vi "command move.vi"(8 "error in (no error)":errorcluster, 9 "uPosition":i32, 10 "Position":i32, 11 "id":i32) -> (0 "error out":errorcluster, 3 "function return":i32)   [LabVIEW 2020, in "libximc.lvlib"]
doc: "result_t XIMC_API command_move (device_t id, int Position, int uPosition);"
uses:
  libximc.lvlib
  libximc.dll
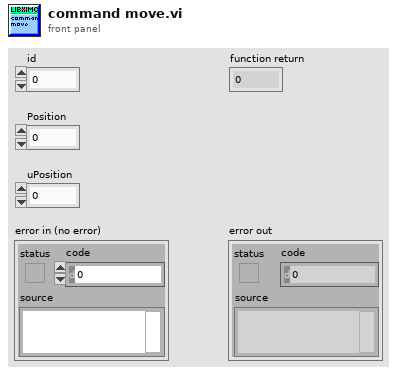
[diagram p1: front panel]
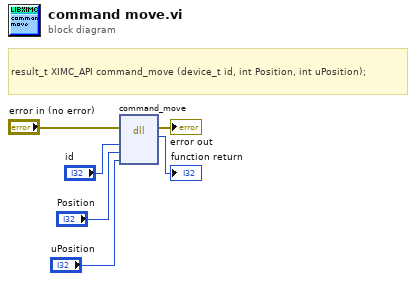
[diagram p0: block diagram]
diagram:
  # "result_t XIMC_API command_move (device_t id, int Position, int uPosition);"
  n1 = dll-call lib="E:/Norway Project/All Hardware/New Microscope/LabVIEW/Stage/libximc.*" fn="command_move"(error in="error in (no error)", "id"="id", "Position"="Position", "uPosition"="uPosition") -> (error out=→"error out":errorcluster, →"function return":i32)  [unwired: 5 in, 1 out]
